vi "Launch Self Update Process.vi"(8 "error in (no error)":errorcluster, 10 "Version":string, 11 "Package Name":string) -> (0 "error out":errorcluster)   [LabVIEW 2022 SP3, in "NIPM_Functions.lvlib"]
uses:
  NIPM_Functions.lvlib
  <vilib>/Utility/error.llb/Trim Whitespace One-Sided.vi
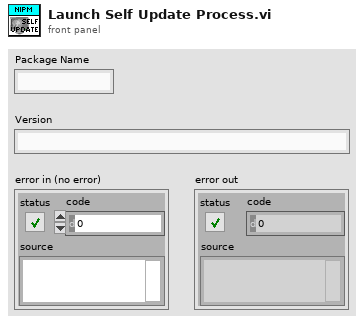
[diagram p1: front panel]
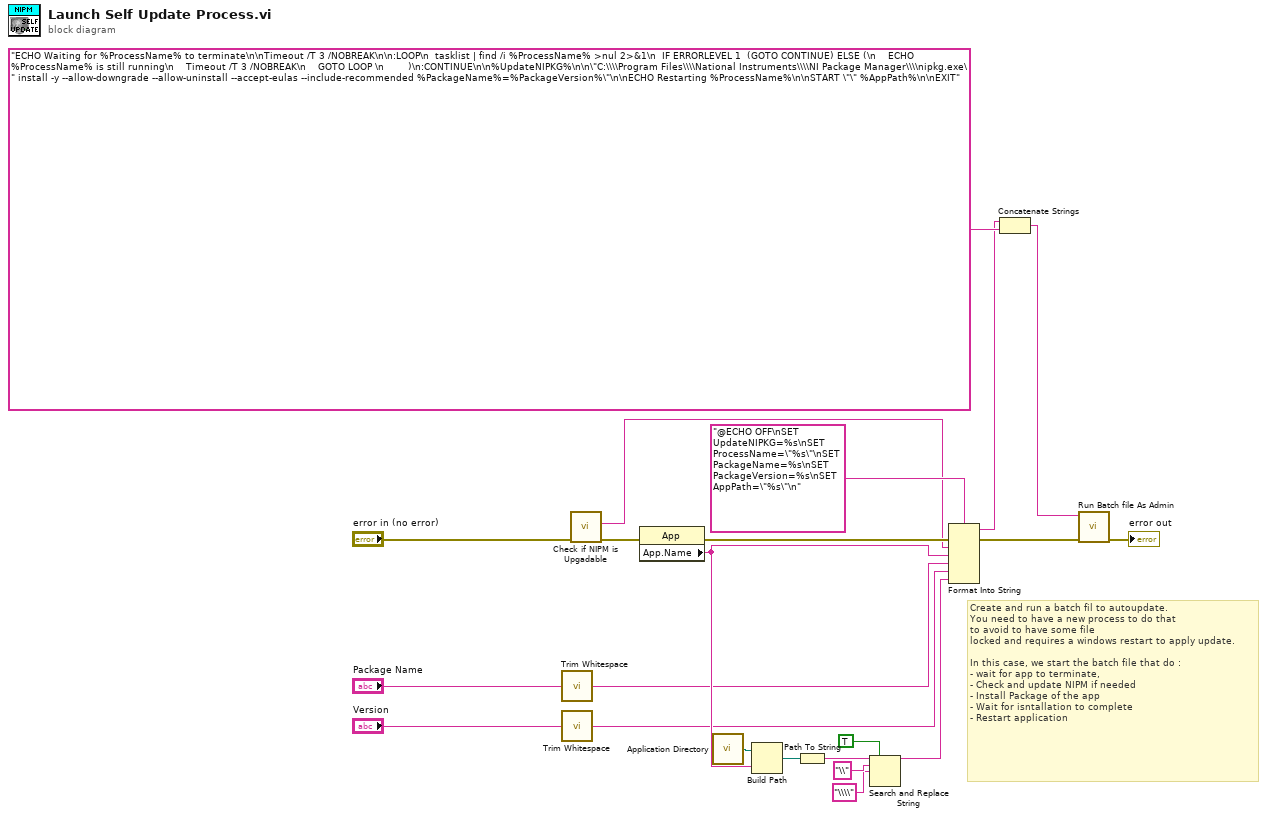
[diagram p0: block diagram]
diagram:
  # "Create and run a batch fil to autoupdate.\nYou need to have a new process to do that \nto avoid to have some file\nlocked and requires a windows restart to apply update.\n\nIn this case, we start the batch file that do :\n- wait for app to terminate,\n- Check and update NIPM if needed\n- Install Package of the app\n- Wait for isntallation to complete\n- Restart application"
  n1 = call <vilib>:"Trim Whitespace.vi"("string"="Package Name") -> ("trimmed string"=w13:string)  [unwired: 1 in]
  n2 = call <vilib>:"Trim Whitespace.vi"("string"="Version") -> ("trimmed string"=w11:string)  [unwired: 1 in]
  n3 = call "Check if NIPM is Upgadable.vi"("error in (no error)"="error in (no error)") -> ("error out"=w5:errorcluster, "Command line"=w3:string)  [unwired: 8 in, 1 out]
  n4 = property class="App"(error in=w5) -> (error out=w22:errorcluster, "App.Name"=w14:string)  [unwired: 1 in, 1 out]
  n5 = call <vilib>:"Application Directory.vi"() -> ("Application Directory"=w17:path)
  n6 = Build Path(base path=w17, name or relative path=w14) -> (appended path=w16:path)
  n7 = Path To String(path=w16) -> (string=w21:string)
  n8 = Search and Replace String(replace all?=TRUE ("replace all? (F)"), input string=w21, search string="\\", replace string="\\\\" ("replace string (\"\")")) -> (result string=w9:string)  [unwired: 4 in, 3 out]
  n9 = Format Into String(format string="@ECHO OFF\nSET UpdateNIPKG=%s\nSET ProcessName=\"%s\"\nSET PackageName=%s\nSET PackageVersion=%s\nSET AppPath=\"%s\"\n", error in=w22, w3, w14, w13, w11, w9) -> (resulting string=w6:string, error out=w2:errorcluster)  [unwired: 1 in]
  n10 = Concatenate Strings(w6, "ECHO Waiting for %ProcessName% to terminate\n\nTimeout /T 3 /NOBREAK\n\n:LOOP\n  tasklist | find /i %ProcessName% >nul 2>&1\n  IF ERRORLEVEL 1  (GOTO CONTINUE) ELSE (\n    ECHO %ProcessName% is still running\n    Timeout /T 3 /NOBREAK\n    GOTO LOOP \n        )\n:CONTINUE\n\n%UpdateNIPKG%\n\n\"C:\\\\Program Files\\\\National Instruments\\\\NI Package Manager\\\\nipkg.exe\" install -y --allow-downgrade --allow-uninstall --accept-eulas --include-recommended %PackageName%=%PackageVersion%\"\n\nECHO Restarting %ProcessName%\n\nSTART \"\" %AppPath%\n\nEXIT" ("command line")) -> (w1:string)
  n11 = call "Run Batch file As Admin.vi"("error in (no error)"=w2, "BAT File Content"=w1) -> ("error out"=→"error out":errorcluster)  [unwired: 9 in]
